vi "Element.vi"(11 "VolatusConfigElement in":refnum<class "VolatusConfigElement.lvclass">) -> (2 "Element":refnum<class "Config Element.lvclass">, 3 "VolatusConfigElement out":refnum<class "VolatusConfigElement.lvclass">)   [LabVIEW 2020, in "VolatusConfig.lvlib" / "VolatusConfigElement.lvclass"]
uses:
  VolatusConfigElement.lvclass
  VolatusConfigElement.lvclass/VolatusConfigElement.ctl
  lv-cdm/CDM-Config/Config Element/Config Element.lvclass
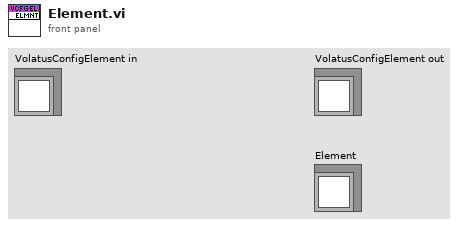
[diagram p1: front panel]
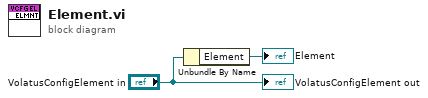
[diagram p0: block diagram]
diagram:
  n1 = Unbundle By Name("VolatusConfigElement in") -> ("Element"=→"Element":refnum<class "Config Element.lvclass">)
  "VolatusConfigElement out" <- "VolatusConfigElement in"
